vi "Const frame basic keyword.vi"() -> (3 "Const frame basic keyword":string[](array[string]))   [LabVIEW 2018, in "Frame Analizer.lvclass"]
uses:
  Frame Analizer.lvclass
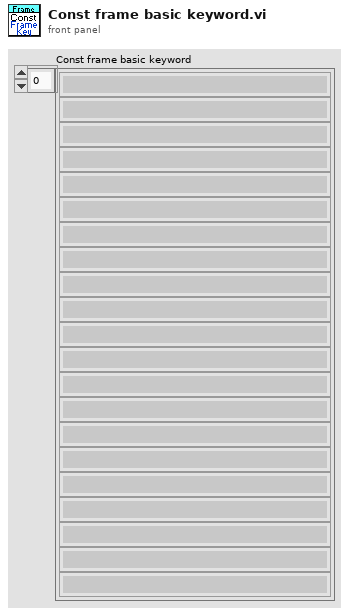
[diagram p1: front panel]
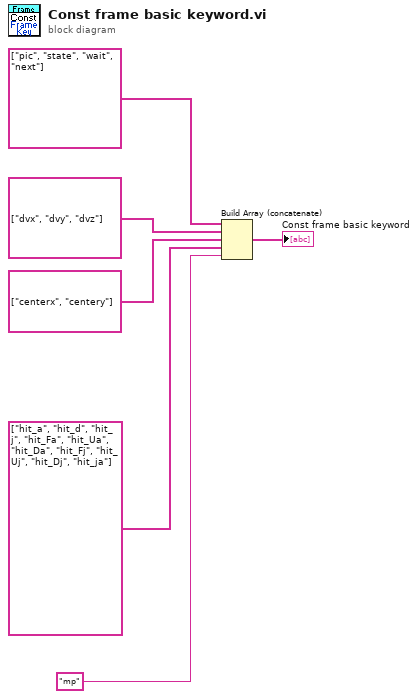
[diagram p0: block diagram]
diagram:
  n1 = Build Array (concatenate)(string[] ["pic", "state", "wait", "next"], string[] ["dvx", "dvy", "dvz"], string[] ["centerx", "centery"], string[] ["hit_a", "hit_d", "hit_j", "hit_Fa", "hit_Ua", "hit_Da", "hit_Fj", "hit_Uj", "hit_Dj", "hit_ja"], "mp") -> (→"Const frame basic keyword":string[])
